vi "Gama.vi"() -> ()   [LabVIEW 2018]
panel:
  out "Gama":dbl
  out "Gama-R":dbl
  in  "Partial Pressure of Water Vapor":dbl
  out "Partial Presure of Water Vapor":dbl(knob) scale=0.0..2.0
  out "Temprature of Humid Air\nKelvin Degree":dbl(slide) scale=273.0..373.0
  out "Tk":dbl
  out "Gama0":dbl
  in  "Tceg":dbl
  out "Temprature of Humid Air\nCentigrade Degree":dbl(slide) scale=0.0..100.0
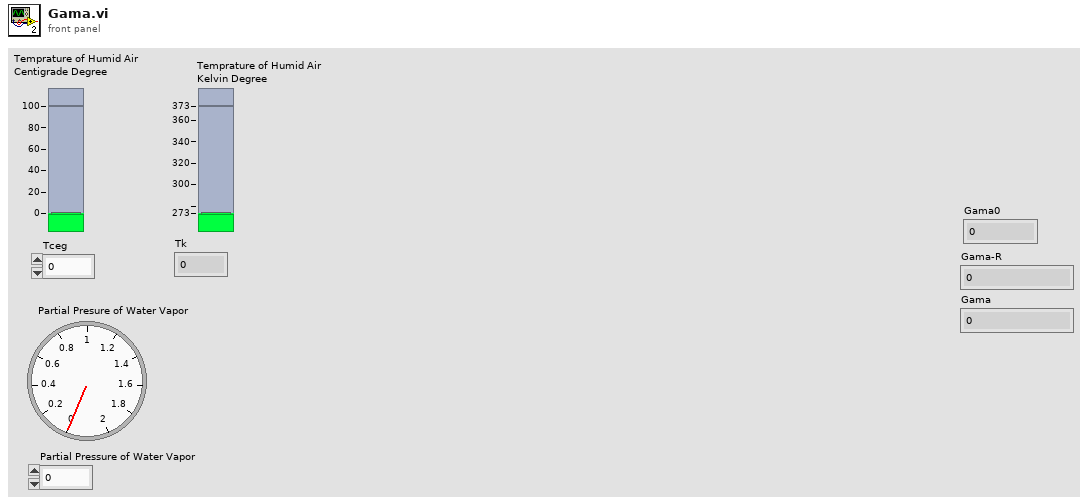
[diagram p1: front panel]
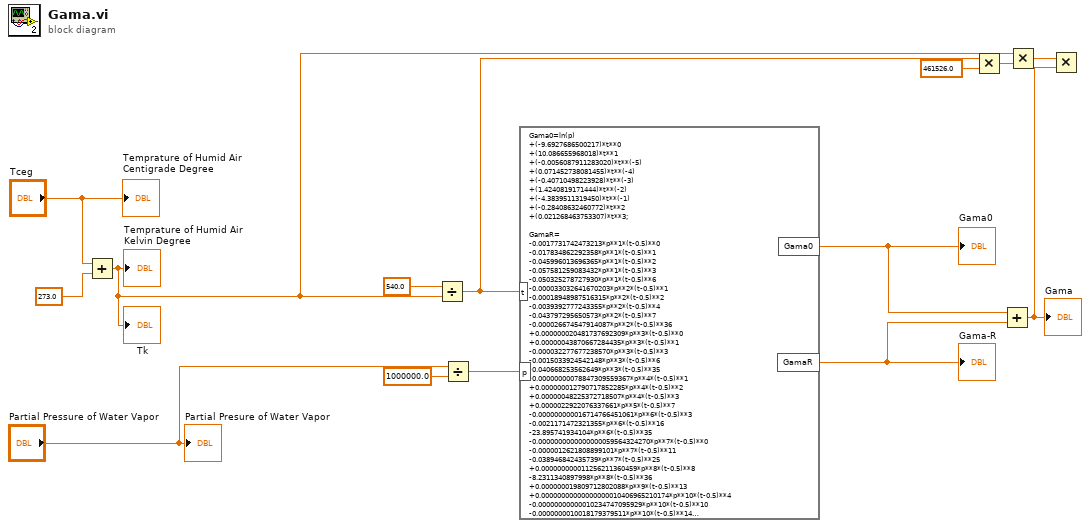
[diagram p0: block diagram]
diagram:
  n1 = Add(x="Tceg", y=273.0) -> (x+y=w3:dbl)
  "Tk" <- w3
  "Temprature of Humid Air\nKelvin Degree" <- w3
  n2 = Divide(x=540.0, y=w3) -> (x/y=w5:dbl)
  n3 = Divide(x="Partial Pressure of Water Vapor", y=1000000.0) -> (x/y=w11:dbl)
  n4 = formula code="Gama0=ln(p)\n+(-9.6927686500217)*t**0\n+(10.086655968018)*t**1\n+(-0.0056087911283020)*t**(-5)\n+(0.071452738081455)*t**(-4)\n+(-0.40710498223928)*t**(-3)\n+(1.4240819171444)*t**(-2)\n+(-4.3839511319450)*t**(-1)\n+(-0.28408632460772)*t**2\n+(0.021268463753307)*t**3;\n\nGamaR=\n-0.0017731742473213*p**1*(t-0.5)**0\n-0.017834862292358*p**1*(t-0.5)**1\n-0.045996013696365*p**1*(t-0.5)**2\n-0.057581259083432*p**1*(t-0.5)**3\n-0.050325278727930*p**1*(t-0.5)**6\n-0.000033032641670203*p**2*(t-0.5)**1\n-0.00018948987516315*p**2*(t-0.5)**2\n-0.0039392777243355*p**2*(t-0.5)**4\n-0.043797295650573*p**2*(t-0.5)**7\n-0.000026674547914087*p**2*(t-0.5)**36\n+0.000000020481737692309*p**3*(t-0.5)**0\n+0.00000043870667284435*p**3*(t-0.5)**1\n-0.000032277677238570*p**3*(t-0.5)**3\n-0.0015033924542148*p**3*(t-0.5)**6\n-0.040668253562649*p**3*(t-0.5)**35\n-0.00000000078847309559367*p**4*(t-0.5)**1\n+0.000000012790717852285*p**4*(t-0.5)**2\n+0.00000048225372718507*p**4*(t-0.5)**3\n+0.0000022922076337661*p**5*(t-0.5)**7\n-0.000000000016714766451061*p**6*(t-0.5)**3\n-0.0021171472321355*p**6*(t-0.5)**16\n-23.895741934104*p**6*(t-0.5)**35\n-0.0000000000000000059564324270*p**7*(t-0.5)**0\n-0.0000012621808899101*p**7*(t-0.5)**11\n-0.038946842435739*p**7*(t-0.5)**25\n+0.000000000011256211360459*p**8*(t-0.5)**8\n-8.2311340897998*p**8*(t-0.5)**36\n+0.000000019809712802088*p**9*(t-0.5)**13\n+0.00000000000000000010406965210174*p**10*(t-0.5)**4\n-0.00000000000010234747095929*p**10*(t-0.5)**10\n-0.0000000010018179379511*p**10*(t-0.5)**14\n-0.000000000080882908646985*p**16*(t-0.5)**29\n+0.10693031879409*p**16*(t-0.5)**50\n-0.33662250574171*p**18*(t-0.5)**57\n+0.00000000000000000000000089185845355421*p**20*(t-0.5)**20\n+0.00000000000030629306876232*p**20*(t-0.5)**35\n-0.42002467698208*10**(-5)*p**20*(t-0.5)**48\n-0.59056029685639*10**(-25)*p**21*(t-0.5)**21\n+0.37826947613457*10**(-5)*p**22*(t-0.5)**53\n-0.12768608934681*10**(-14)*p**23*(t-0.5)**39\n+0.73087610595061*10**(-28)*p**24*(t-0.5)**26\n+0.55414715350778*10**(-16)*p**24*(t-0.5)**40\n-0.94369707241210*10**(-6)*p**24*(t-0.5)**58;"("t"=w5, "p"=w11) -> ("Gama0"=w8:dbl, "GamaR"=w7:dbl)
  "Gama0" <- w8
  "Gama-R" <- w7
  n5 = Multiply(x=w5, y=461526.0) -> (x*y=w4:dbl)
  n6 = Add(x=w8, y=w7) -> (x+y=w1:dbl)
  "Gama" <- w1
  n7 = Multiply(x=w3, y=w4) -> (x*y=w2:dbl)
  n8 = Multiply(x=w2, y=w1) -> ()  [unwired: 1 out]
  "Temprature of Humid Air\nCentigrade Degree" <- "Tceg"
  "Partial Presure of Water Vapor" <- "Partial Pressure of Water Vapor"
